vi "Range Conversion.vi"(6 "New Min":dbl, 7 "New Max":dbl, 8 "Current Min":dbl, 10 "Input Value":dbl, 11 "Current Max":dbl) -> (2 "Scaled Output":dbl)   [LabVIEW 2017]
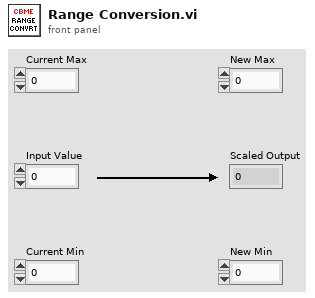
[diagram p1: front panel]
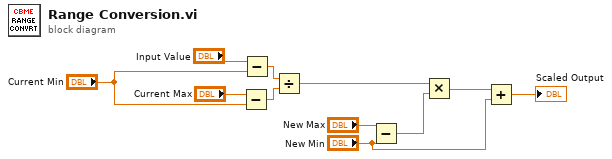
[diagram p0: block diagram]
diagram:
  n1 = Subtract(x="Current Max", y="Current Min") -> (x-y=w7:dbl)
  n2 = Subtract(x="Input Value", y="Current Min") -> (x-y=w8:dbl)
  n3 = Divide(x=w8, y=w7) -> (x/y=w4:dbl)
  n4 = Subtract(x="New Max", y="New Min") -> (x-y=w5:dbl)
  n5 = Multiply(x=w4, y=w5) -> (x*y=w3:dbl)
  n6 = Add(x=w3, y="New Min") -> (x+y=→"Scaled Output":dbl)
